vi "Get LV Server Class Ancestry.vi"(4 "error in":errorcluster, 6 "Use Localized (T)":bool=TRUE, 7 "Class Name":string="Invoke") -> (0 "error out":errorcluster, 2 "Ancestor Class Names":string[](array[string]), 3 "Ancestor Class ID Strings":string[](array[string]))   [LabVIEW 2025, in "XNode Support.lvlib"]
uses:
  XNode Support.lvlib
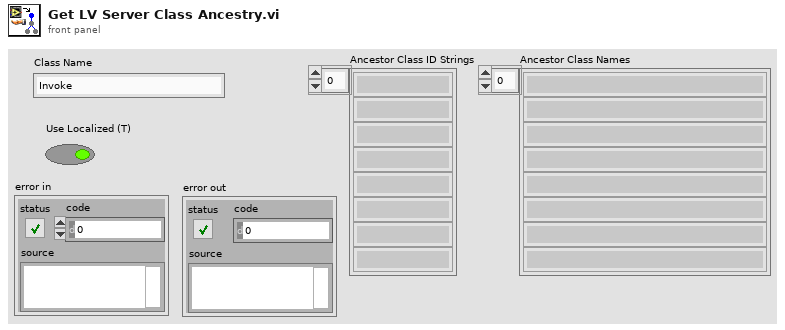
[diagram p1: front panel]
types:
  T1 = typedef "ASC_ArrayOfUniqueIDStringParentIDStringName.ctl" = T2[]
  T2 = typedef "ASC_UniqueIDStringParentIDStringName.ctl" = cluster{"Unique ID string":string, "Parent ID string":string, "Class Name (unlocalized)":string, "Class Name (localized)":string}
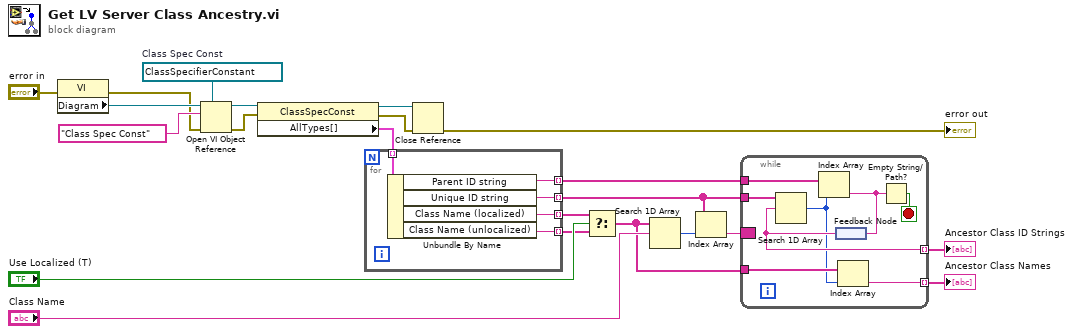
[diagram p0: block diagram]
diagram:
  w7 = refnum<vi> refnum  # Class Spec Const
  n1 = property class="VI"(error in="error in") -> (error out=w4:errorcluster, "Diagram"=w5:refnum<vi>)  [unwired: 1 in, 1 out]
  n2 = Open VI Object Reference(7:w7, 8:w4, 10:"Class Spec Const" ("name/order"), 11:w5) -> (0:w2:errorcluster, 3:w3:refnum<vi>)
  n3 = property class="ClassSpecConst"(reference=w3, error in=w2) -> (reference out=w1:refnum<vi>, error out=w11:errorcluster, "AllTypes[]"=w12:T1)
  n4 = for {
    tunnel: w12 -> [w23] mode=indexing
    tunnel: [w27] -> w18 mode=indexing
    tunnel: [w26] -> w17 mode=indexing
    tunnel: [w25] -> w20 mode=indexing
    tunnel: [w24] -> w19 mode=indexing
    n5 = Unbundle By Name(w23) -> ("Parent ID string"=w27:string, "Unique ID string"=w26:string, "Class Name (localized)"=w25:string, "Class Name (unlocalized)"=w24:string)
  }
  n6 = Close Reference(reference=w1, error in (no error)=w11) -> (error out=→"error out":errorcluster)
  n7 = Select(t=w20, s="Use Localized (T)", f=w19) -> (s? t:f=w14:string[])
  n8 = Search 1D Array(1D array=w14, element="Class Name") -> (index of element=w16:i32)  [unwired: 1 in]
  n9 = Index Array(array=w17, index=w16) -> (element=w8:string)
  n10 = while {
    tunnel: w18 -> [w35]
    tunnel: w17 -> [w33]
    tunnel: [w32] -> w15 mode=indexing
    tunnel: w14 -> [w31]
    tunnel: [w29] -> w13 mode=indexing
    border: w8 -> [_]
    stop <- w34 stop-if-true
    n11 = feedback #1() -> (w32:string)
    n12 = Search 1D Array(1D array=w33, element=w32) -> (index of element=w30:i32)  [unwired: 1 in]
    n13 = Index Array(array=w35, index=w30) -> (element=w28:string)
    n14 = feedback-in #1(w28) -> ()
    n15 = Index Array(array=w31, index=w30) -> (element=w29:string)
    n16 = Empty String/Path?(string/path=w28) -> (empty?=w34:bool)
  }
  "Ancestor Class ID Strings" <- w15
  "Ancestor Class Names" <- w13
